vi "Dual Mux.vi"() -> ()   [LabVIEW 2019]
uses:
  <vilib>/myRIO/Instrument Drivers/Onboard IO/I2C/typedefs/I2C User Configuration.ctl
  <vilib>/myRIO/Instrument Drivers/Onboard IO/I2C/typedefs/I2C Transfer Rate.ctl
  <vilib>/myRIO/Instrument Drivers/Onboard IO/I2C/typedefs/I2C Reference.ctl
  <vilib>/myRIO/Common/Instrument Driver Framework/Utilities/typedefs/myRIO Generic Hardware Reference.ctl
  <vilib>/myRIO/Common/Instrument Driver Framework/Utilities/typedefs/Hardware Version Enum.ctl
  <vilib>/myRIO/Common/Instrument Driver Framework/Utilities/typedefs/myRIO v1.0 Reference.ctl
  <vilib>/myRIO/Common/Instrument Driver Framework/Utilities/typedefs/Generic FPGA Reference.ctl
  <vilib>/myRIO/Common/Instrument Driver Framework/myRIO v1.0/I2C/typedefs/I2C Channels Enum.ctl
  <vilib>/myRIO/Instrument Drivers/Onboard IO/I2C/typedefs/I2C Configuration.ctl
  <vilib>/userDefined/High Color/nirio_resource_hc.ctl
  <vilib>/Platform/TimedLoop/XDataNode/timing_clust.ctl
  <vilib>/Platform/TimedLoop/XDataNode/nitl_modes.ctl
  <vilib>/Platform/TimedLoop/XDataNode/wakeup.ctl
  <vilib>/myRIO/Common/Instrument Driver Framework/Utilities/vis/Is FPGA Ref Available.vi
  <vilib>/myRIO/Common/Instrument Driver Framework/myRIO v1.0/I2C/vis/myRIO v1.1 Open I2C.vi
  <vilib>/myRIO/Instrument Drivers/Onboard IO/I2C/vis/Configure.vi
  <vilib>/myRIO/Instrument Drivers/Onboard IO/I2C/vis/Write.vi
  <vilib>/myRIO/Instrument Drivers/Onboard IO/I2C/vis/Write Read.vi
  <vilib>/myRIO/Common/Instrument Driver Framework/Utilities/vis/Validate Channels.vi
  <vilib>/myRIO/Common/Instrument Driver Framework/myRIO v1.0/I2C/vis/myRIO v1.0 Reserve I2C.vi
  <vilib>/myRIO/Common/Instrument Driver Framework/myRIO v1.0/UART/vis/myRIO v1.0 Close UART.vi
  <vilib>/myRIO/Common/Instrument Driver Framework/myRIO v1.0/I2C/vis/myRIO v1.0 Build MUX Configuration I2C.vi
  <vilib>/myRIO/Common/Instrument Driver Framework/myRIO v1.0/Resource Manager/vis/myRIO v1.0 Reserve Channel List.vi
  <vilib>/myRIO/Common/Instrument Driver Framework/myRIO v1.0/Resource Manager/vis/myRIO v1.0 Create Configuration List.vi
  <vilib>/myRIO/Common/Instrument Driver Framework/myRIO v1.0/Resource Manager/vis/myRIO v1.0 Reserve Channel.vi
  <vilib>/myRIO/Common/Instrument Driver Framework/myRIO v1.0/Resource Manager/vis/myRIO v1.0 Unreserve Channel.vi
  <vilib>/myRIO/Common/Instrument Driver Framework/myRIO v1.0/Resource Manager/vis/myRIO v1.0 Build Mutex Name.vi
  <vilib>/Utility/VariantDataType/GetNumericInfo.vi
  <vilib>/Utility/error.llb/Error Cluster From Error Code.vi
  <vilib>/myRIO/Common/Instrument Driver Framework/myRIO v1.0/myRIO v1.1 Open.vi
  <vilib>/myRIO/Common/Instrument Driver Framework/Utilities/vis/IO Manager.vi
  <vilib>/myRIO/Common/Instrument Driver Framework/Utilities/vis/Configuration Manager.vi
  <vilib>/myRIO/Common/Instrument Driver Framework/myRIO v1.0/Resource Manager/vis/myRIO v1.0 Configure IO.vi
  <vilib>/myRIO/Common/Instrument Driver Framework/myRIO v1.0/myRIO v1.0 Close.vi
  <vilib>/myRIO/Common/Instrument Driver Framework/myRIO v1.0/I2C/vis/myRIO v1.0 Configure I2C.vi
  <vilib>/myRIO/Common/Instrument Driver Framework/myRIO v1.0/I2C/vis/myRIO v1.0 Write I2C.vi
  <vilib>/myRIO/Common/Instrument Driver Framework/myRIO v1.0/I2C/vis/myRIO v1.0 Read I2C.vi
  <vilib>/Utility/file.llb/Write Delimited Spreadsheet (DBL).vi
  <vilib>/myRIO/Common/Instrument Driver Framework/Utilities/vis/FPGA Ref Manager.vi
  <vilib>/myRIO/Common/Instrument Driver Framework/myRIO v1.0/myRIO v1.0 Reset FPGA.vi
  <vilib>/myRIO/Common/Instrument Driver Framework/myRIO v1.0/IRQ/vis/myRIO v1.0 IRQ Info FGV.vi
  <vilib>/myRIO/Common/Instrument Driver Framework/myRIO v1.0/IRQ/vis/myRIO v1.0 Timer IRQ Info FGV.vi
  <vilib>/myRIO/Common/Instrument Driver Framework/myRIO v1.0/IRQ/vis/myRIO v1.0 ISR Agent.vi
  <vilib>/myRIO/Instrument Drivers/Utilities/vis/Reset Index.vi
  <vilib>/myRIO/Common/Instrument Driver Framework/myRIO v1.0/Resource Manager/vis/myRIO v1.0 Block Write Resource Manager.vi
  <vilib>/myRIO/Express VI/Onboard IO/I2C/I2C Express VI.xnode
  <vilib>/myRIO/Instrument Drivers/Onboard IO/I2C/vis/myRIO I2C Open.xnode
  <vilib>/platform/TimedLoop/XDataNode/XDataNode.xnode
  <vilib>/myRIO/Instrument Drivers/Onboard IO/I2C/I2C.lvlib
  <vilib>/Platform/TimedLoop/XDataNode/XDNodeRunTimeDep.lvlib
  <vilib>/myRIO/Instrument Drivers/Utilities/Utilities.lvlib
panel:
  in  "file path (dialog if empty)":path
  out "MUX 2":cluster{dbl, dbl, dbl}(graph) caption="Waveform Chart"
  in  "stop":bool
  out "MUX 1":cluster{dbl, dbl, dbl}(graph) caption="Waveform Chart"
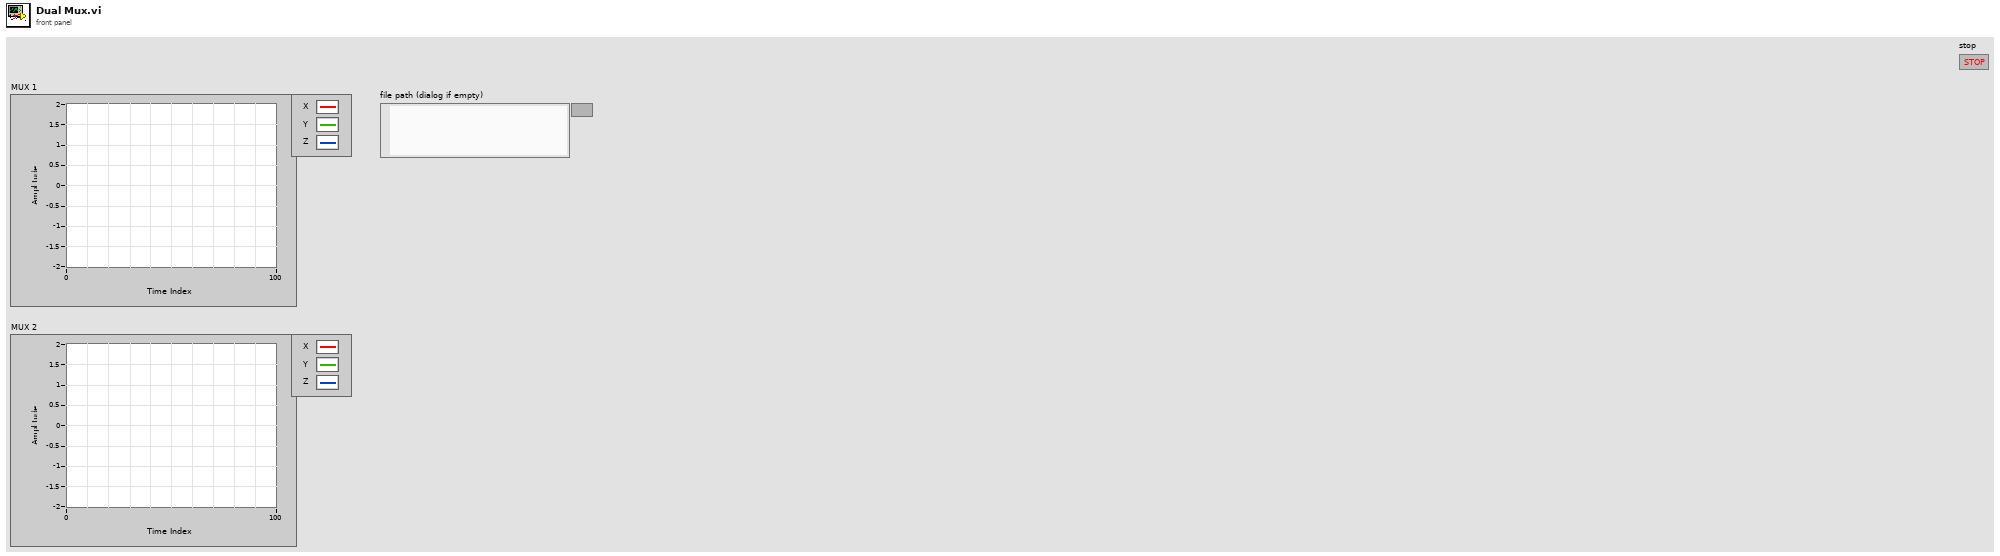
[diagram p1: front panel]
types:
  T1 = typedef "I2C.lvlib/I2C Reference.ctl" = cluster{"myRIO Reference":T2, "I2C Channels Enum":T6, "I2C Configuration":T7}
  T2 = typedef "myRIO Generic Hardware Reference.ctl" = cluster{"myRIO Model":T3, "myRIO Hardware Reference":T4}
  T3 = typedef "Hardware Version Enum.ctl" = enum16{"Unknown", "myRIO-1900", "myRIO-1950", "roboRIO", "NI ELVIS RIO CM", "ELVIS III"}
  T4 = typedef "myRIO v1.0 Reference.ctl" = cluster{"Generic FPGA Reference":T5, "Allow multiple opens":bool}
  T5 = typedef "Generic FPGA Reference.ctl" = refnum<k20>
  T6 = typedef "I2C Channels Enum.ctl" = enum16{"Not Connected", "A/I2C", "B/I2C", "I2C/I2C"}
  T7 = typedef "I2C.lvlib/I2C Configuration.ctl" = cluster{"I2C Transfer Rate":T8}
  T8 = typedef "I2C.lvlib/I2C Transfer Rate.ctl" = enum16{"Standard mode (100 kbps)", "Fast mode (400 kbps)"}
  T9 = typedef "I2C.lvlib/I2C User Configuration.ctl" = cluster{"I2C Transfer Rate":T8}
  T10 = typedef "nirio_resource_hc.ctl" = tag
  T11 = typedef "XDNodeRunTimeDep.lvlib/timing_clust.ctl" = cluster{"Expected End [f-1]":u64, "Actual End [f-1]":u64, "Finished Late? [f-1]":bool, "Expected End [i-1]":u64, "Actual End [i-1]":u64, "Finished Late? [i-1]":bool, "Expected Start [i]":u64, "Actual Start [i]":u64, "Expected Start [f]":u64, "Actual Start [f]":u64, "Source Name":string, "Structure Name":string, "Period":i64, "Deadline":i64, "Offset":i64, "Start":i64, "Priority":i32, "Timeout":i32, "Mode":T12, "Wakeup Reason":T13, "Error":errorcluster, "Source Type":string, "Secondary Source Type":string, "Global End Time":u64, "Global Start Time":u64, "Frame Duration":u64, "Iteration Duration":u64, "Assigned CPU":i32, "I/O Scan Engine Mode":u32}
  T12 = typedef "XDNodeRunTimeDep.lvlib/nitl_modes.ctl" = enum32{"No Change", "Process missed periods, maintain original phase", "Discard missed periods, maintain original phase", "Process missed periods, ignore original phase", "Discard missed periods, ignore original phase"}
  T13 = typedef "XDNodeRunTimeDep.lvlib/wakeup.ctl" = enum32{"Normal", "Aborted", "Asynchronous wakeup", "Timing source error", "Timed loop error", "Timeout"}
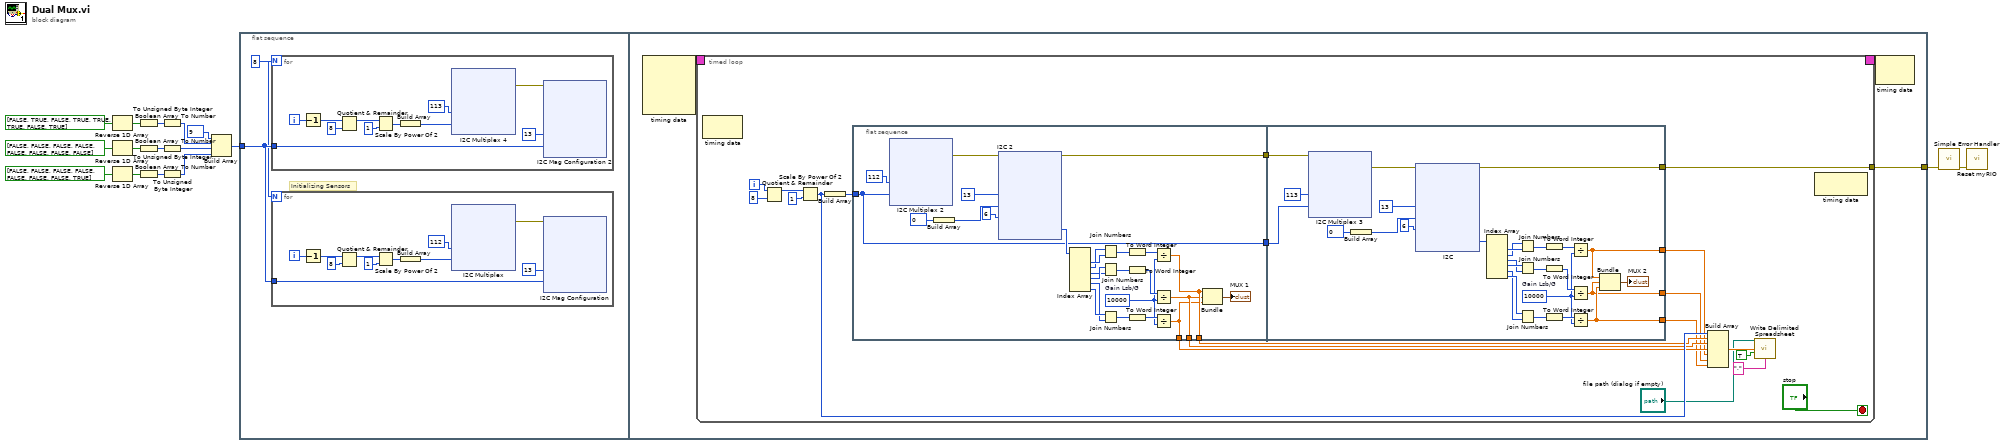
[diagram p0: block diagram]
diagram:
  n1 = Reverse 1D Array(array=bool[] [FALSE, TRUE, FALSE, TRUE, TRUE, TRUE, FALSE, TRUE]) -> (reversed array=w15:bool[])
  n2 = Reverse 1D Array(array=bool[] [FALSE, FALSE, FALSE, FALSE, FALSE, FALSE, FALSE, FALSE]) -> (reversed array=w14:bool[])
  n3 = Reverse 1D Array(array=bool[] [FALSE, FALSE, FALSE, FALSE, FALSE, FALSE, FALSE, TRUE]) -> (reversed array=w12:bool[])
  n4 = Boolean Array To Number(Boolean array=w15) -> (number=w9:u32)
  n5 = Boolean Array To Number(Boolean array=w14) -> (number=w8:u32)
  n6 = Boolean Array To Number(Boolean array=w12) -> (number=w7:u32)
  n7 = To Unsigned Byte Integer(number=w9) -> (unsigned 8bit integer=w6:u8)
  n8 = To Unsigned Byte Integer(number=w8) -> (unsigned 8bit integer=w5:u8)
  n9 = To Unsigned Byte Integer(number=w7) -> (unsigned 8bit integer=w4:u8)
  n10 = Build Array(u8 9 ("address"), w6, w5, w4) -> (w3:u8[])
  n11 = flat-sequence {
    tunnel: w3 -> [w18]
    tunnel: [w193] -> w2
    frame #0 {
      w17 = 8
      # "Initializing Sensors"
      n12 = for {
        N: w17 -> [_]
        tunnel: w18 -> [w26]
        i -> [w20]
        n13 = Decrement(x=w20) -> (x-1=w19:i32)
        n14 = Quotient & Remainder(x=w19, y=8) -> (x-y*floor(x/y)=w21:i32)  [unwired: 1 out]
        n15 = Scale By Power Of 2(n=w21, x=1) -> (x*2^n=w23:i32)
        n16 = Build Array(w23) -> (w29:i32[])
        n17 = xnode "I2C Multiplex 4"("Slave Address (7-bit)"=u8 113, "Bytes to Write"=w29) -> ("error out"=w28:errorcluster)  [unwired: 1 in]
        n18 = xnode "I2C Mag Configuration 2"("Slave Address (7-bit)"=u8 13, "Bytes to Write"=w26, "error in (no error)"=w28) -> ()  [unwired: 1 out]
      }
      n19 = for {
        N: w17 -> [_]
        tunnel: w18 -> [w113]
        i -> [w107]
        n20 = Decrement(x=w107) -> (x-1=w106:i32)
        n21 = Quotient & Remainder(x=w106, y=8) -> (x-y*floor(x/y)=w108:i32)  [unwired: 1 out]
        n22 = Scale By Power Of 2(n=w108, x=1) -> (x*2^n=w110:i32)
        n23 = Build Array(w110) -> (w116:i32[])
        n24 = xnode "I2C Multiplex"("Slave Address (7-bit)"=u8 112, "Bytes to Write"=w116) -> ("error out"=w115:errorcluster)  [unwired: 1 in]
        n25 = xnode "I2C Mag Configuration"("Slave Address (7-bit)"=u8 13, "Bytes to Write"=w113, "error in (no error)"=w115) -> ()  [unwired: 1 out]
      }
    }
    frame #1 {
      n26 = node-c288() -> (w195:T11)  [unwired: 4 in]
      n27 = timed-loop {
        timing: w195 -> [_]
        timing-out: [_] -> w194
        tunnel: [w208] -> w193
        i -> [w212]
        stop <- "stop" stop-if-true
        n28 = node-c288() -> ()  [unwired: 1 in, 1 out]
        n29 = Quotient & Remainder(x=w212, y=8) -> (x-y*floor(x/y)=w209:i32)  [unwired: 1 out]
        n30 = Scale By Power Of 2(n=w209, x=1) -> (x*2^n=w205:i32)
        n31 = Build Array(w205) -> (w213:i32[])
        n32 = flat-sequence {
          tunnel: w213 -> [w221]
          tunnel: [w221] -> w210
          tunnel: [w219] -> w207
          tunnel: [w218] -> w204
          tunnel: [w217] -> w203
          tunnel: [w216] -> w202
          tunnel: w210 -> [w326]
          tunnel: w207 -> [w323]
          tunnel: [w324] -> w208
          tunnel: [w322] -> w201
          tunnel: [w321] -> w200
          tunnel: [w320] -> w199
          frame #0 {
            w231 = i16 10000  # Gain Lsb/G
            n33 = xnode "I2C Multiplex 2"("Slave Address (7-bit)"=u8 112, "Bytes to Write"=w221) -> ("error out"=w220:errorcluster)  [unwired: 1 in]
            n34 = Build Array(u8 0) -> (w235:u8[])
            n35 = xnode "I2C 2"("Slave Address (7-bit)"=u8 13, "Bytes to Write"=w235, "Byte Count"=u32 6, "error in (no error)"=w220) -> ("Bytes Read"=w238:u8[], "error out"=w219:errorcluster)
            n36 = Index Array(array=w238) -> (element #1=w229:u8, element #2=w228:u8, element #3=w226:u8, element #4=w227:u8, element #5=w224:u8, element #6=w225:u8)  [unwired: 6 in]
            n37 = Join Numbers(hi=w228, lo=w229) -> ((hi.lo)=w241:u16)
            n38 = Join Numbers(hi=w227, lo=w226) -> ((hi.lo)=w239:u16)
            n39 = Join Numbers(hi=w225, lo=w224) -> ((hi.lo)=w240:u16)
            n40 = To Word Integer(number=w241) -> (16bit integer=w234:i16)
            n41 = To Word Integer(number=w239) -> (16bit integer=w233:i16)
            n42 = To Word Integer(number=w240) -> (16bit integer=w232:i16)
            n43 = Divide(x=w234, y=w231) -> (x/y=w218:dbl)
            n44 = Divide(x=w233, y=w231) -> (x/y=w217:dbl)
            n45 = Divide(x=w232, y=w231) -> (x/y=w216:dbl)
            n46 = Bundle(w218, w217, w216) -> (→"MUX 1":cluster{dbl, dbl, dbl})  [unwired: 1 in]
          }
          frame #1 {
            w336 = i16 10000  # Gain Lsb/G
            n47 = xnode "I2C Multiplex 3"("Slave Address (7-bit)"=u8 113, "Bytes to Write"=w326, "error in (no error)"=w323) -> ("error out"=w325:errorcluster)
            n48 = Build Array(u8 0) -> (w340:u8[])
            n49 = xnode "I2C"("Slave Address (7-bit)"=u8 13, "Bytes to Write"=w340, "Byte Count"=u32 6, "error in (no error)"=w325) -> ("Bytes Read"=w343:u8[], "error out"=w324:errorcluster)
            n50 = Index Array(array=w343) -> (element #1=w334:u8, element #2=w333:u8, element #3=w331:u8, element #4=w332:u8, element #5=w329:u8, element #6=w330:u8)  [unwired: 6 in]
            n51 = Join Numbers(hi=w333, lo=w334) -> ((hi.lo)=w346:u16)
            n52 = Join Numbers(hi=w332, lo=w331) -> ((hi.lo)=w344:u16)
            n53 = Join Numbers(hi=w330, lo=w329) -> ((hi.lo)=w345:u16)
            n54 = To Word Integer(number=w346) -> (16bit integer=w339:i16)
            n55 = To Word Integer(number=w344) -> (16bit integer=w338:i16)
            n56 = To Word Integer(number=w345) -> (16bit integer=w337:i16)
            n57 = Divide(x=w339, y=w336) -> (x/y=w322:dbl)
            n58 = Divide(x=w338, y=w336) -> (x/y=w320:dbl)
            n59 = Divide(x=w337, y=w336) -> (x/y=w321:dbl)
            n60 = Bundle(w322, w320, w321) -> (→"MUX 2":cluster{dbl, dbl, dbl})  [unwired: 1 in]
          }
        }
        n61 = Build Array(w205, w204, w203, w202, w201, w199, w200) -> (w206:dbl[])
        n62 = call-poly <vilib>:"Write Delimited Spreadsheet.vi"("file path (dialog if empty)"="file path (dialog if empty)", "1D data"=w206, "append to file? (new file:F)"=TRUE, "delimiter (\\t)"="," ("delimiter (\\t)")) -> ()  [unwired: 10 in, 2 out]
        n63 = node-c288() -> ()  [unwired: 1 in, 1 out]
      }
      n64 = node-c288(w194) -> ()  [unwired: 1 out]
    }
  }
  n65 = call <vilib>:"Simple Error Handler.vi"("error in (no error)"=w2) -> ("error out"=w1:errorcluster)  [unwired: 4 in, 4 out]
  n66 = call <vilib>:"Reset myRIO.vi"("error in (no error)"=w1) -> ()  [unwired: 10 in, 1 out]
